vi "RPC Method hello_hi.vi"(8 "error in (no error)":errorcluster, 11 "OOP Server in":refnum<class "Simple_server.lvclass">) -> (0 "error out":errorcluster, 3 "OOP Server out":refnum<class "Simple_server.lvclass">)   [LabVIEW 2019, in "Simple_server.lvlib" / "Simple_server.lvclass"]
uses:
  Simple_server.lvclass
  Simple_server.lvclass/Simple_server.ctl
  RPC Messages/simpleMgsReply/simpleMgsReply_Data.ctl
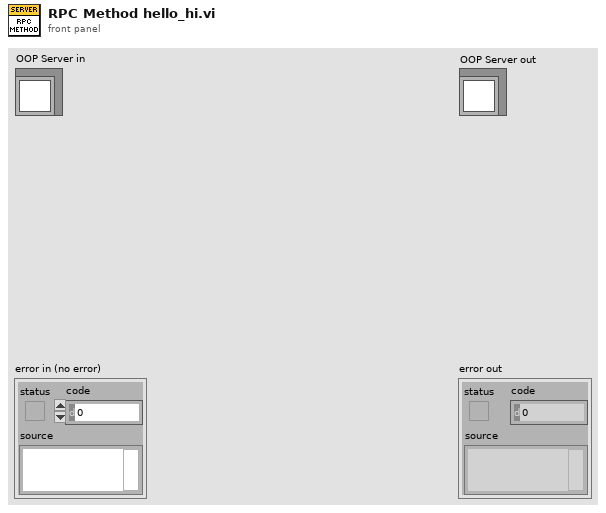
[diagram p1: front panel]
types:
  T1 = typedef "Simple_server.lvlib/Simple_server.lvclass/simpleMgsReply_Data.ctl" = cluster{"hello":string}
  T2 = typedef "Simple_server.lvlib/Simple_server.lvclass/Server Internal UEs.ctl" = cluster{"hello_hi Internal UE":refnum<user-event>}
  T3 = typedef "Simple_server.lvlib/Simple_server.lvclass/Server gRPC UEs.ctl" = cluster{"hello_hi gRPC UE":refnum<user-event>}
  T4 = typedef "gprc-lvsupport-release.lvlib/grpcId.ctl" = u64
  T5 = typedef "Simple_server.lvlib/Simple_server.lvclass/simpleMsgReq_Data.ctl" = cluster{"name":string}
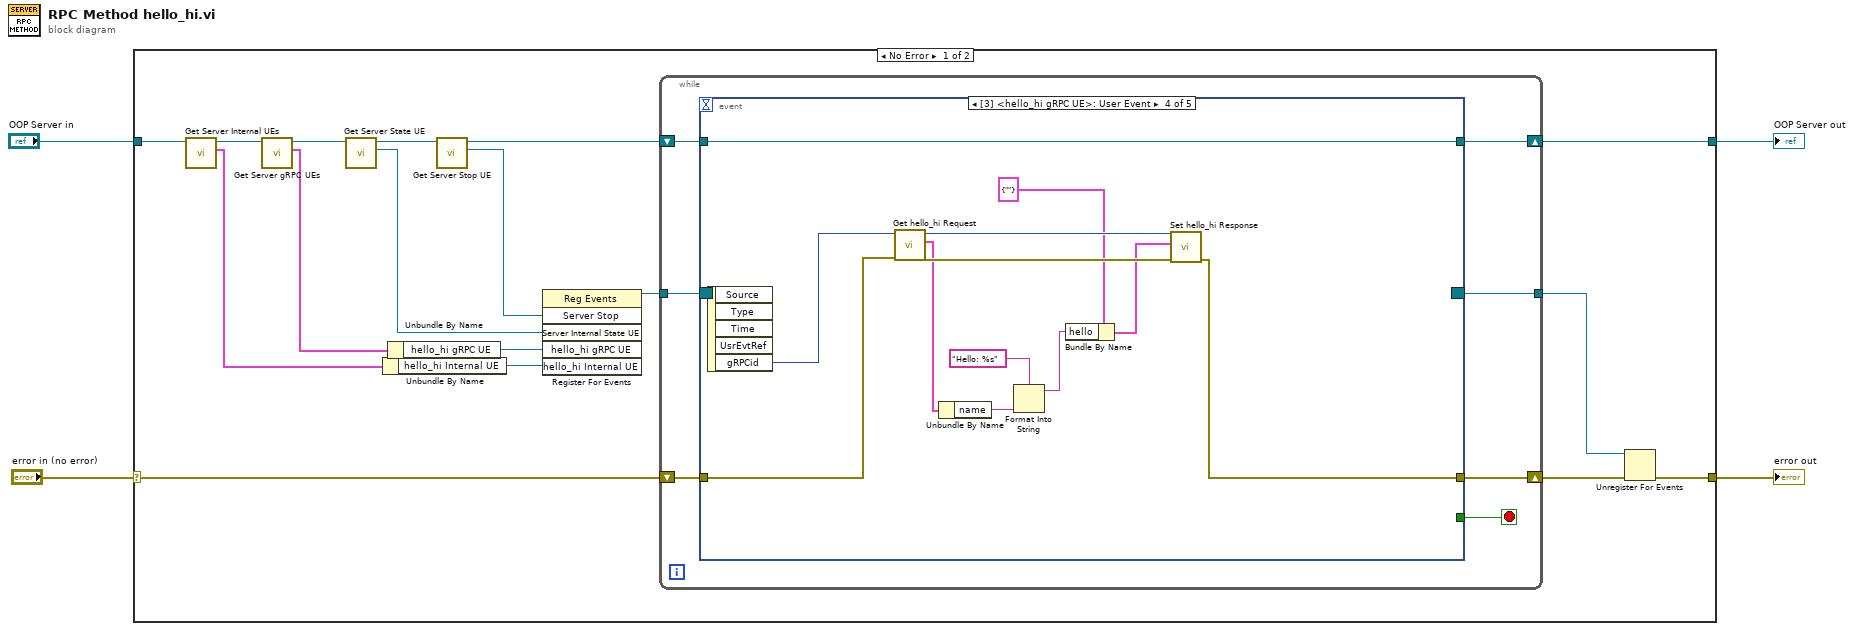
[diagram p0: block diagram]
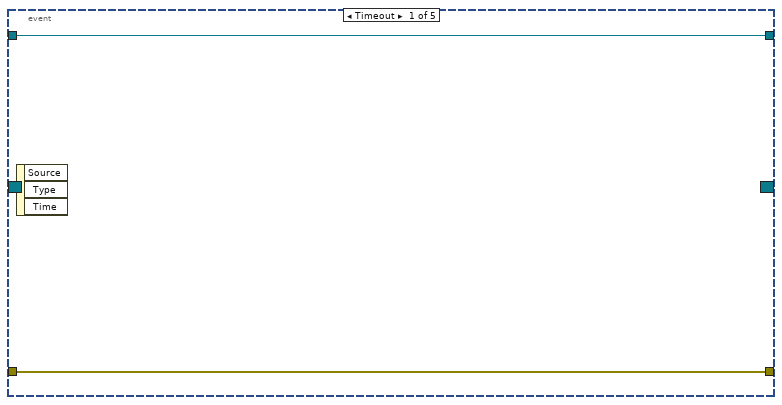
[diagram p2: hidden frame]
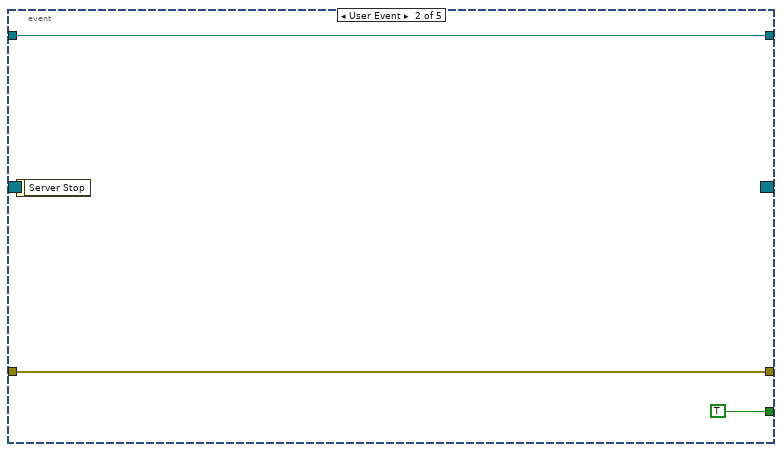
[diagram p3: hidden frame]
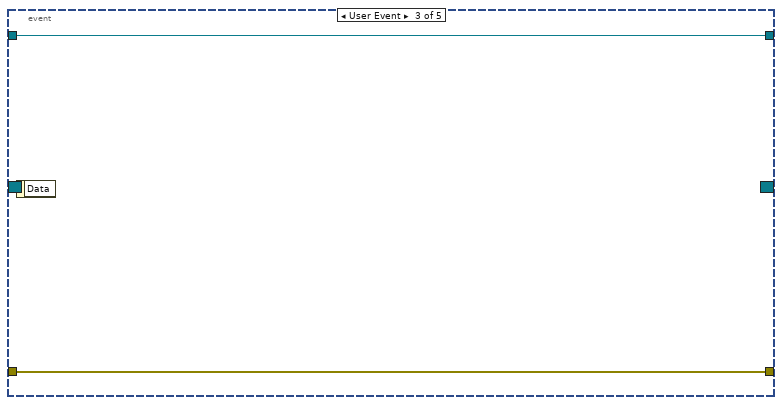
[diagram p4: hidden frame]
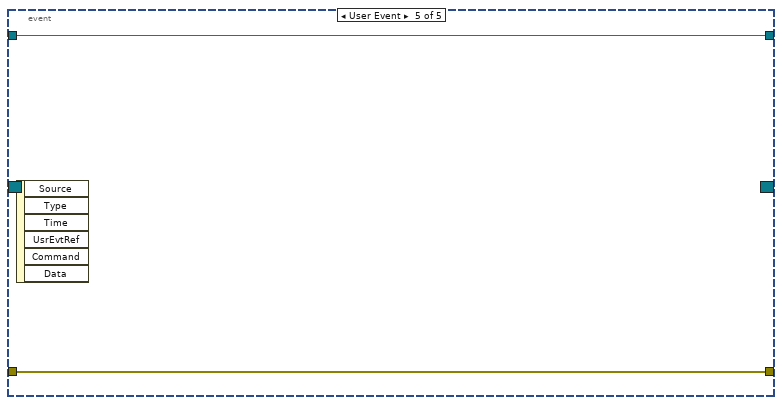
[diagram p5: hidden frame]
diagram:
  n1 = case shown="No Error" "error in (no error)" {
    selector: "error in (no error)" -> [w17 w51]
    tunnel: [w15 w51] -> w3
    tunnel: "OOP Server in" -> [w19 w50]
    tunnel: [w5 w50] -> w1
    frame No Error {
      n2 = call "Get Server Internal UEs.vi"("OOP Server in"=w19) -> ("Server Internal UEs"=w11:T2, "OOP Server out"=w18:refnum<class "Simple_server.lvclass">)  [unwired: 9 in]
      n3 = call "Get Server gRPC UEs.vi"("OOP Server in"=w18) -> ("Server RPC Methods"=w13:T3, "OOP Server out"=w8:refnum<class "Simple_server.lvclass">)  [unwired: 9 in]
      n4 = call "Get Server State UE.vi"("Template Server in"=w8) -> ("Server Internal State UE"=w6:refnum<user-event>, "Template Server out"=w7:refnum<class "Simple_server.lvclass">)  [unwired: 9 in]
      n5 = Unbundle By Name ("Unbundle Internal UE")(w11) -> ("hello_hi Internal UE"=w10:refnum<user-event>)
      n6 = Unbundle By Name ("Unbundle gRPC UE")(w13) -> ("hello_hi gRPC UE"=w12:refnum<user-event>)
      n7 = call "Get Server Stop UE.vi"("OOP Server in"=w7) -> ("Server Stop"=w21:refnum<user-event>, "OOP Server out"=w9:refnum<class "Simple_server.lvclass">)  [unwired: 9 in]
      n8 = register-events(w21, w6, w12, w10) -> (reference out=w20:refnum<event-registration>)  [unwired: 2 in, 1 out]
      n9 = while {
        tunnel: w20 -> [w28]
        tunnel: [w24] -> w14
        shift-right: [w25] -> w16
        shift-left: w17 -> [w26]
        shift-right: [w22] -> w5
        shift-left: w9 -> [w23]
        stop <- w27 stop-if-true
        n10 = event "RPC Method Event Structure" shown="[3] <hello_hi gRPC UE>: User Event" {
          selector: w28 -> [_ _ _ _ _]
          dyn-events: [_ _ _ _ _] -> w24
          timeout: _ -> [_ _ _ _ _]
          tunnel: [_ TRUE _ _ _] -> w27
          tunnel: w26 -> [w30 w32 w35 w42 w49]
          tunnel: [w30 w32 w35 w43 w49] -> w25
          tunnel: w23 -> [w29 w31 w34 w47 w48]
          tunnel: [w29 w31 w34 w47 w48] -> w22
          event Timeout {
            n11 = event-data() -> ()  [unwired: 1 in, 3 out]
          }
          event User Event {
            n12 = event-data() -> ()  [unwired: 1 in, 1 out]
          }
          event User Event {
            n13 = event-data() -> ()  [unwired: 1 in, 1 out]
          }
          event User Event {
            n14 = event-data() -> ("gRPCid"=w46:T4)  [unwired: 1 in, 4 out]
            n15 = call "Get hello_hi Request.vi"("error in (no error)"=w42, "gRPCid in"=w46) -> ("error out"=w44:errorcluster, "Message Data"=w41:T5, "gRPCid out"=w45:T4)  [unwired: 7 in]
            n16 = Unbundle By Name(w41) -> ("name"=w37:string)
            n17 = Format Into String(format string="Hello: %s", w37) -> (resulting string=w36:string)  [unwired: 2 in, 1 out]
            n18 = Bundle By Name(cluster=T1 {"hello"=""} ("Message Data"), "hello"=w36) -> (w39:T1)
            n19 = call "Set hello_hi Response.vi"("error in (no error)"=w44, "Message Data"=w39, "gRPCid in"=w45) -> ("error out"=w43:errorcluster)  [unwired: 8 in]
          }
          event User Event {
            n20 = event-data() -> ()  [unwired: 1 in, 6 out]
          }
        }
      }
      n21 = Unregister For Events(event registration refnum=w14, error in=w16) -> (error out=w15:errorcluster)
    }
    frame Error {
    }
  }
  "error out" <- w3
  "OOP Server out" <- w1
